vi "get data interface information.vi"(11 "Temperature Controller Logic runtime in":refnum<class "Temperature Controller Logic runtime.lvclass">) -> (2 "data type defs":T1, 3 "Temperature Controller Logic runtime out":refnum<class "Temperature Controller Logic runtime.lvclass">)   [LabVIEW 2013, in "Temperature Controller Logic runtime.lvclass"]
uses:
  Temperature Controller Logic runtime.lvclass
  <vilib>/NI/Tag Bus Data Framework/fixed module parent/module/execution/data cluster type definition.ctl
  output user data.ctl
  parameter user data.ctl
  result user data.ctl
  input user data.ctl
  <vilib>/NI/Tag Bus Data Framework/fixed module parent/module/execution/fixed channel runtime.lvclass
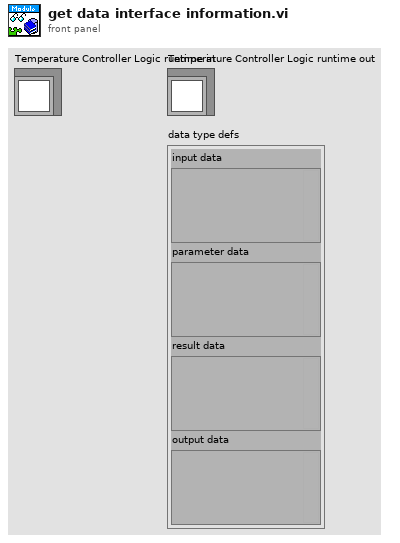
[diagram p1: front panel]
types:
  T1 = typedef "fixed channel runtime.lvclass/data cluster type definition.ctl" = cluster{"input data":variant, "parameter data":variant, "result data":variant, "output data":variant}
  T2 = typedef "Temperature Controller Logic runtime.lvclass/input user data.ctl" = cluster{"placeholder":sgl}
  T3 = typedef "Temperature Controller Logic runtime.lvclass/result user data.ctl" = cluster{"fan":dbl, "lamp":dbl}
  T4 = typedef "Temperature Controller Logic runtime.lvclass/parameter user data.ctl" = cluster{"Temperature":dbl, "setpoint":dbl, "output range high":dbl, "output range low":dbl, "Kc":dbl, "Ti":dbl, "Td":dbl, "Fan on?":bool}
  T5 = typedef "Temperature Controller Logic runtime.lvclass/output user data.ctl" = cluster{"placeholder":sgl}
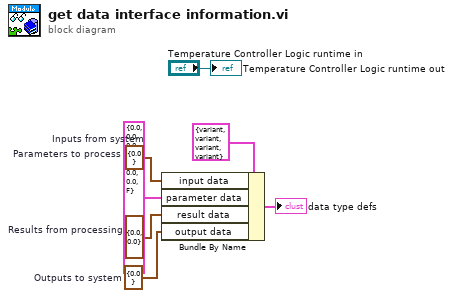
[diagram p0: block diagram]
diagram:
  w1 = T2 {"placeholder"=0.0}  # Inputs from system
  w3 = T3 {"fan"=0.0, "lamp"=0.0}  # Results from processing
  w2 = T4 {"Temperature"=0.0, "setpoint"=0.0, "output range high"=0.0, "output range low"=0.0, "Kc"=0.0, "Ti"=0.0, "Td"=0.0, "Fan on?"=FALSE}  # Parameters to process
  w4 = T5 {"placeholder"=0.0}  # Outputs to system
  n1 = Bundle By Name(cluster=T1 {"input data"=variant, "parameter data"=variant, "result data"=variant, "output data"=variant} ("data type defs"), "input data"=w1, "parameter data"=w2, "result data"=w3, "output data"=w4) -> (→"data type defs":T1)
  "Temperature Controller Logic runtime out" <- "Temperature Controller Logic runtime in"
